vi "sub_nmea_checksum.vi"(10 "nmea checksum":string, 11 "nmea raw":string) -> (2 "checksum_val":u8, 3 "checksum":bool)   [LabVIEW 2019]
panel:
  out "sum":u8 format="%02x"
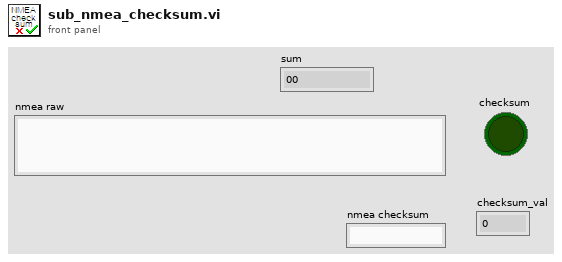
[diagram p1: front panel]
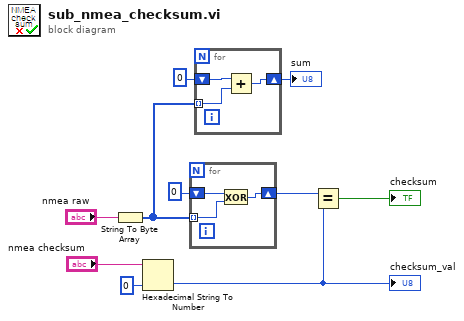
[diagram p0: block diagram]
diagram:
  n1 = String To Byte Array(string="nmea raw") -> (unsigned byte array=w2:u8[])
  n2 = Hexadecimal String To Number(string="nmea checksum", default (0uL)=u8 0 ("default (0 U32)")) -> (number=w10:u8)  [unwired: 1 in, 1 out]
  "checksum_val" <- w10
  n3 = for {
    tunnel: w2 -> [w12] mode=indexing
    shift-right: [w11] -> w5
    shift-left: u8 0 ("sum") -> [w13]
    n4 = Exclusive Or(1:w12, 2:w13) -> (0:w11:u8)
  }
  n5 = for {
    tunnel: w2 -> [w15] mode=indexing
    shift-right: [w14] -> w1
    shift-left: u8 0 ("sum") -> [w16]
    n6 = Add(x=w16, y=w15) -> (x+y=w14:u8)
  }
  "sum" <- w1
  n7 = Equal?(x=w5, y=w10) -> (x = y?=→"checksum":bool)
